vi "FPGA Main Default.vi"() -> ()   [LabVIEW 2015]
doc: "The myRIO v1.1 FPGA Shipping Personality. This personality contains support for:\n- 2 Analog Input Interrupt channel\n- 4 Digital Input Interrupt channel\n- 1 Timer\n- 1 Accelerometer\n- 1 Button\n- 4 LED\n- 10 Analog Input channels with 1 Sample\n- 6 Analog Output channels with 1 Sample\n- 40 Digital I/O channels with 1 Sample\n- 2 I2C channels\n- 4 Encoder channels\n- 6 PWM channels\n- 2 SPI channels"
uses:
  Sub VIs/Utilities/Start Boolean.ctl
  <vilib>/Platform/TimedLoop/XDataNode/timing_clust.ctl
  <vilib>/Platform/TimedLoop/XDataNode/nitl_modes.ctl
  <vilib>/Platform/TimedLoop/XDataNode/wakeup.ctl
  <vilib>/rvi/Emulation/niFpgaGetClockAttributes.vi
  <vilib>/rvi/Emulation/niFpgaSctlEmulationGetInTimedLoop.vi
  <vilib>/rvi/Emulation/niFpgaEmulationReportErrorSimple.vi
  <vilib>/rvi/eio/common/nirviEmuTemplateMethod_errors.vi
  <vilib>/rvi/Emulation/niFpgaCriticalErrorInLSC.vi
  <vilib>/rvi/Emulation/niFpgaProcessEmulError.vi
  <vilib>/rvi/Emulation/niFpgaEmulationIsFPGAContextNoSignature.vi
  <vilib>/rvi/errors/niFpgaSetErrorForExecOnDevCompSimple.vi
  <vilib>/rvi/eio/common/nirviEmuReportErrorAndStop.vi
  <vilib>/rvi/DataTransferAndStorage/Container/Common/niFpgaContainerGetUniqueNameForEmu.vi
  <vilib>/rvi/FIFO/Fifo_Resource/nirvififoEmulationSetSize.vi
  <vilib>/rvi/FIFO/Fifo_Resource/nirviFifoEmulationQueueMgr.vi
  <instcachedir>/0/nirviFifoEmulationQueueMgr_E5CAEC123FF24DC58D834DCA3CDAA9B5.lvgen/nirviFifoEmulationQueueMgr_E5CAEC123FF24DC58D834DCA3CDAA9B5_002.vi
  <vilib>/rvi/FIFO/Fifo_Resource/nirvififoEmulationDetermineInputValidOut.vi
  <vilib>/rvi/FIFO/Fifo_Resource/nirvififoEmulationCreateLock.vi
  <vilib>/rvi/FIFO/Fifo_Resource/nirvififoEmulationObtainLock.vi
  <vilib>/rvi/FIFO/Fifo_Resource/nirvififoEmulationReleaseLock.vi
  <vilib>/rvi/occurrence/nirviWaitOnOccurrenceBase.vi
  <vilib>/rvi/errors/nirviReportUnexpectedCaseInternalError.vi
  <vilib>/rvi/errors/nirviReportUnexpectedCaseInternalError (U32).vi
  <vilib>/Utility/error.llb/Clear Errors.vi
  <vilib>/rvi/DataTransferAndStorage/Container/Common/niFpgaContainerSetEmuInfo.vi
  <vilib>/eio/EIONode/EIONode.xnode
  <vilib>/rvi/DataTransferAndStorage/Container/XNode/niFpgaContainer.xnode
  <vilib>/rvi/FIFO/Fifo_Resource/nirvififoEmulationWrite.vi
  <vilib>/rvi/FIFO/Fifo_Resource/nirvififoEmulationRead.vi
  <vilib>/Platform/TimedLoop/XDataNode/XDataNode.xnode
  <vilib>/rvi/LocalResourceManager/LocalResourceManager.xnode
  <vilib>/Platform/TimedLoop/XDataNode/XDNodeRunTimeDep.lvlib
panel:
  in  "AO.A_0.VAL":u16
  in  "AO.A_1.VAL":u16
  in  "AO.B_0.VAL":u16
  in  "AO.B_1.VAL":u16
  out "AI.B_3.VAL":u16
  out "AI.B_2.VAL":u16
  out "AI.B_1.VAL":u16
  out "AI.B_0.VAL":u16
  out "AI.A_3.VAL":u16
  out "AI.A_2.VAL":u16
  out "AI.A_1.VAL":u16
  out "AI.A_0.VAL":u16
  out "DIO.B_7:0.IN":u8 format="%08b"
  in  "DIO.B_7:0.DIR":u8 format="%08b"
  in  "DIO.B_7:0.OUT":u8 format="%08b"
  in  "PWM.A_2.CS":u8=1
  in  "PWM.A_2.CNFG":u8=4
  out "PWM.A_2.CNTR":u16
  in  "PWM.A_2.MAX":u16=39999
  in  "PWM.A_2.CMP":u16=20000
  in  "PWM.A_1.CS":u8=1
  in  "PWM.A_1.CNFG":u8=4
  out "PWM.A_1.CNTR":u16
  in  "PWM.A_1.MAX":u16=39999
  in  "PWM.A_1.CMP":u16=20000
  in  "PWM.A_0.CS":u8=1
  in  "PWM.A_0.CNFG":u8=4
  out "PWM.A_0.CNTR":u16
  in  "PWM.A_0.CMP":u16=20000
  in  "PWM.A_0.MAX":u16=39999
  in  "SPI.A.DATO":u16
  out "SPI.A.DATI":u16
  in  "SPI.A.CNFG":u16=112
  in  "SPI.A.CNT":u16=19
  in  "SPI.B.CNT":u16=19
  in  "SPI.B.CNFG":u16=112 format="%0.0f"
  out "SPI.B.DATI":u16
  in  "SPI.B.DATO":u16
  in  "ENC.A.CNFG":u8 format="%08b"
  in  "ENC.B.CNFG":u8 format="%08b"
  out "ENC.A.CNTR":u32
  out "ENC.B.CNTR":u32
  out "ENC.A.STAT":u8 format="%08b"
  out "ENC.B.STAT":u8 format="%08b"
  in  "SPI.A.GO":T1
  out "SPI.A.STAT":u8 format="%08b"
  in  "SPI.B.GO":T1
  out "SPI.B.STAT":u8 format="%08b"
  out "I2C.B.STAT":u8 format="%08b"
  in  "I2C.B.CNTL":u8 format="%08b"
  out "I2C.A.STAT":u8 format="%08b"
  in  "I2C.A.CNTL":u8 format="%08b"
  in  "I2C.B.CNTR":u8=213
  in  "I2C.B.ADDR":u8 format="%08.0f"
  out "I2C.B.DATI":u8
  in  "I2C.B.DATO":u8
  in  "I2C.A.CNTR":u8=213
  in  "I2C.A.ADDR":u8 format="%08b"
  out "I2C.A.DATI":u8
  in  "I2C.A.DATO":u8
  in  "I2C.B.CNFG":u8=1 format="%08b"
  in  "I2C.A.CNFG":u8=1 format="%08b"
  in  "I2C.A.GO":T1
  in  "I2C.B.GO":T1
  out "SYS.AI.RDY":bool
  out "SYS.RDY":bool
  in  "PWM.B_2.CS":u8=1
  in  "PWM.B_2.CNFG":u8=4
  out "PWM.B_2.CNTR":u16
  in  "PWM.B_2.MAX":u16=39999
  in  "PWM.B_2.CMP":u16=20000
  in  "PWM.B_1.CS":u8=1
  in  "PWM.B_1.CNFG":u8=4
  out "PWM.B_1.CNTR":u16
  in  "PWM.B_1.MAX":u16=39999
  in  "PWM.B_1.CMP":u16=20000
  in  "PWM.B_0.CS":u8=1
  in  "PWM.B_0.CNFG":u8=4
  out "PWM.B_0.CNTR":u16
  in  "PWM.B_0.MAX":u16=39999
  in  "PWM.B_0.CMP":u16=20000
  out "DIO.A_7:0.IN":u8 format="%08b"
  in  "DIO.A_7:0.OUT":u8 format="%08b"
  in  "DIO.A_7:0.DIR":u8 format="%08b"
  in  "SYS.SELECTB":u8 format="%08b"
  in  "SYS.SELECTA":u8 format="%08b"
  out "DIO.A_15:8.IN":u8 format="%08b"
  in  "DIO.A_15:8.OUT":u8 format="%08b"
  in  "DIO.A_15:8.DIR":u8 format="%08b"
  out "DIO.B_15:8.IN":u8 format="%08b"
  in  "DIO.B_15:8.DIR":u8 format="%08b"
  in  "DIO.B_15:8.OUT":u8 format="%08b"
  in  "AO.SYS.GO":T1
  out "ACC.X.VAL":u16
  out "ACC.Y.VAL":u16
  out "SYS.ACC.RDY":bool
  out "ACC.Z.VAL":u16
  in  "DO.LED3:0":u8 format="%04b"
  out "DI.BTN":u8 format="%08b"
  out "AO.SYS.STAT":bool
  in  "IRQ.AI_A_3:0.CNFG":u8 format="%.0b"
  in  "IRQ.AI_A_0.THRESHOLD":u16
  in  "IRQ.AI_A_1.THRESHOLD":u16
  in  "IRQ.AI_A_0.NO":u8
  in  "IRQ.AI_A_1.NO":u8
  in  "IRQ.DIO_A_7:0.ENA":u8 format="%08b"
  in  "IRQ.DIO_A_7:0.RISE":u8 format="%08b"
  in  "IRQ.DIO_A_7:0.FALL":u8 format="%08b"
  in  "IRQ.DIO_A_0.NO":u8
  in  "IRQ.DIO_A_1.NO":u8
  in  "IRQ.DIO_A_2.NO":u8
  in  "IRQ.DIO_A_3.NO":u8
  in  "IRQ.DIO_A_3.CNT":u32
  in  "IRQ.DIO_A_2.CNT":u32
  in  "IRQ.DIO_A_1.CNT":u32
  in  "IRQ.DIO_A_0.CNT":u32
  in  "IRQ.AI_A_1.HYSTERESIS":u16=17
  in  "IRQ.TIMER.WRITE":u32
  in  "IRQ.TIMER.SETTIME":T1
  out "IRQ.TIMER.READ":u32
  in  "SPI.A.IRQ.NO":u8=15
  in  "SPI.B.IRQ.NO":u8=15
  in  "IRQ.AI_A_0.HYSTERESIS":u16=17
  in  "IRQ.DI_BTN.ENA":bool
  in  "IRQ.DI_BTN.RISE":bool
  in  "IRQ.DI_BTN.FALL":bool
  in  "IRQ.DI_BTN.CNT":u32
  in  "IRQ.DI_BTN.NO":u8
  # "System"
  # "Onboard Devices"
  # "Connector A"
  # "Connector B"
  # "Accelerometer"
  # "Analog Input"
  # "Analog Output"
  # "Digital I/O"
  # "PWM"
  # "SPI Master"
  # "Analog Input"
  # "Analog Output"
  # "Digital I/O"
  # "PWM"
  # "SPI Master"
  # "IO Configuration"
  # "IO Configuration"
  # "Buttons & LEDs"
  # "Analog Interrupt"
  # "Digital Interrupt"
  # "Encoders"
  # "Encoders"
  # "Button Interrupt"
  # "I2C Master"
  # "I2C Master"
  # "Timer Interrupt"
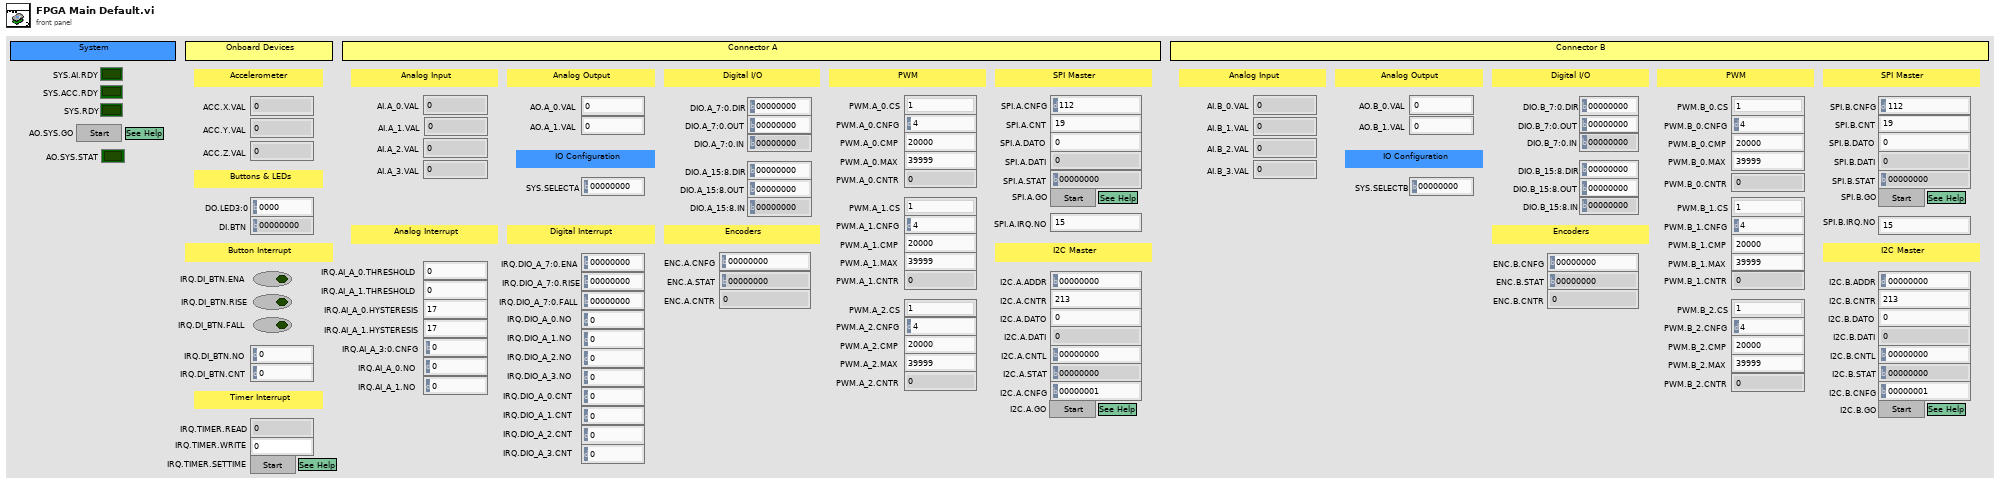
[diagram p1: front panel]
types:
  T1 = typedef "Start Boolean.ctl" = bool
  T2 = typedef "XDNodeRunTimeDep.lvlib/timing_clust.ctl" = cluster{"Expected End [f-1]":u64, "Actual End [f-1]":u64, "Finished Late? [f-1]":bool, "Expected End [i-1]":u64, "Actual End [i-1]":u64, "Finished Late? [i-1]":bool, "Expected Start [i]":u64, "Actual Start [i]":u64, "Expected Start [f]":u64, "Actual Start [f]":u64, "Source Name":string, "Structure Name":string, "Period":i64, "Deadline":i64, "Offset":i64, "Start":i64, "Priority":i32, "Timeout":i32, "Mode":T3, "Wakeup Reason":T4, "Error":errorcluster, "Source Type":string, "Secondary Source Type":string, "Global End Time":u64, "Global Start Time":u64, "Frame Duration":u64, "Iteration Duration":u64, "Assigned CPU":i32, "I/O Scan Engine Mode":u32}
  T3 = typedef "XDNodeRunTimeDep.lvlib/nitl_modes.ctl" = enum32{"No Change", "Process missed periods, maintain original phase", "Discard missed periods, maintain original phase", "Process missed periods, ignore original phase", "Discard missed periods, ignore original phase"}
  T4 = typedef "XDNodeRunTimeDep.lvlib/wakeup.ctl" = enum32{"Normal", "Aborted", "Asynchronous wakeup", "Timing source error", "Timed loop error", "Timeout"}
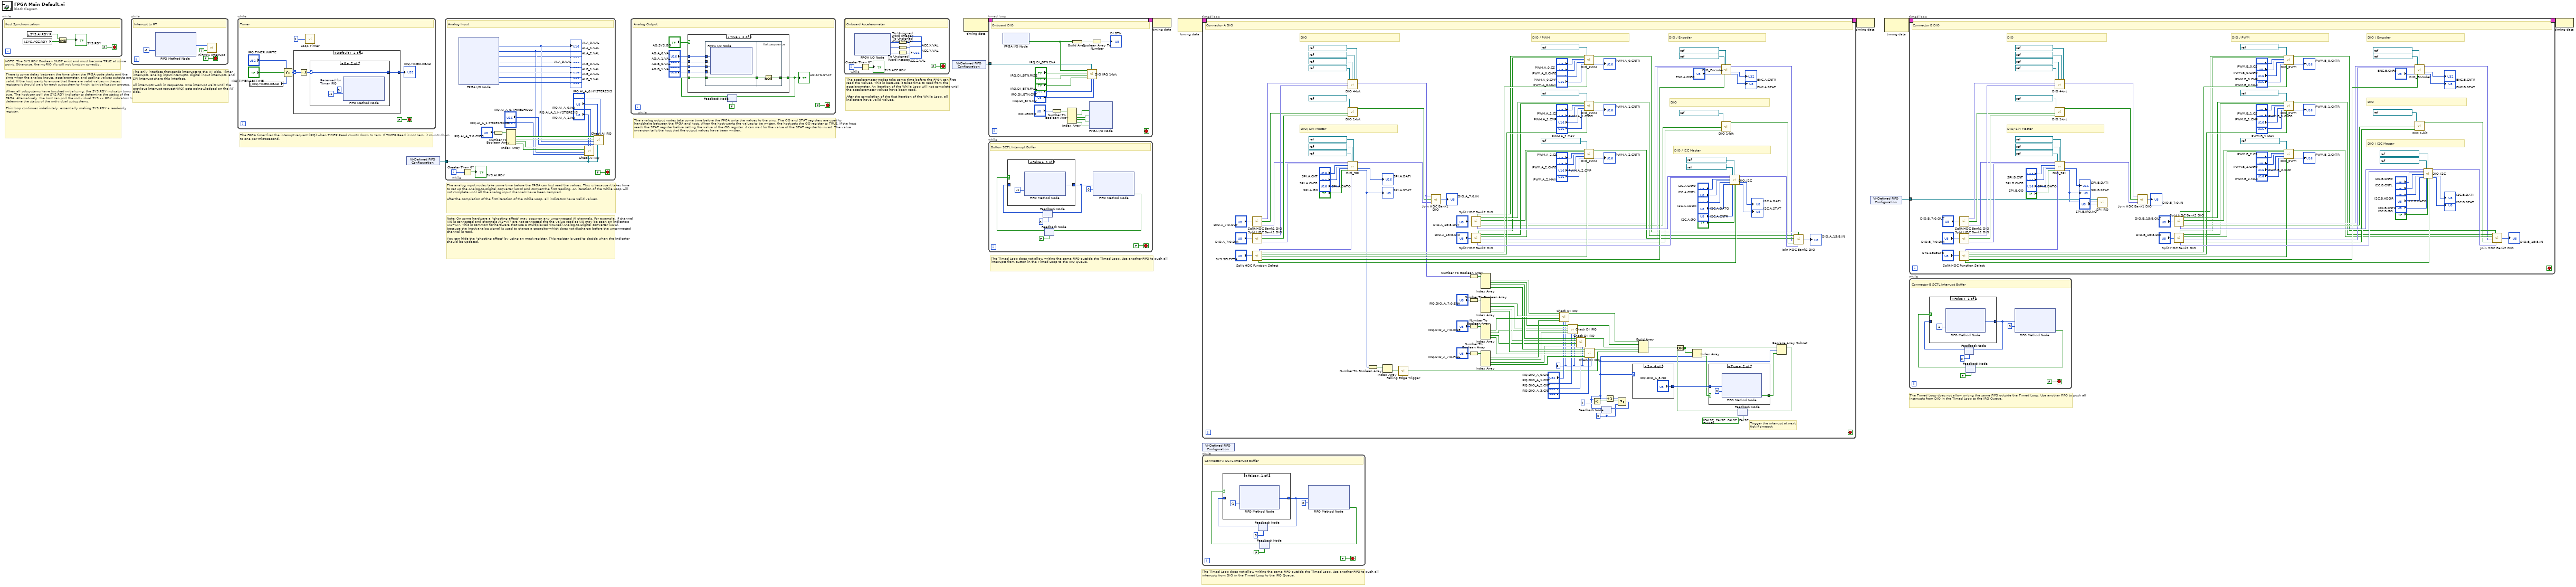
[diagram p0: block diagram]
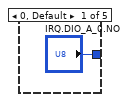
[diagram p9: hidden frame]
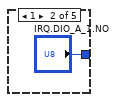
[diagram p10: hidden frame]
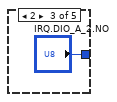
[diagram p11: hidden frame]
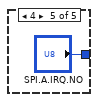
[diagram p12: hidden frame]
diagram:
  # "The Timed Loop does not allow writing the same FIFO outside the Timed Loop. Use another FIFO to push all interrupts from DIO in the Timed Loop to the IRQ Queue."
  # "The Timed Loop does not allow writing the same FIFO outside the Timed Loop. Use another FIFO to push all interrupts from DIO in the Timed Loop to the IRQ Queue."
  # "The Timed Loop does not allow writing the same FIFO outside the Timed Loop. Use another FIFO to push all interrupts from Button in the Timed Loop to the IRQ Queue."
  # "The accelerometer nodes take some time before the FPGA can first read the values. This is because it takes time to read from the accelerometer. An iteration of the While Loop will not complete until the accelerometer values have been read.\n\nAfter the completion of the first iteration of the While Loop, all indicators have valid values."
  # "The analog output nodes take some time before the FPGA write the values to the pins. The GO and STAT registers are used to handshake between the FPGA and host. When the host wants the values to be written, the host sets the GO register to TRUE. If the host reads the STAT register before setting the value of the GO register, it can wait for the value of the STAT register to invert. The value inversion tells the host that the output values have been written."
  # "The analog input nodes take some time before the FPGA can first read the values. This is because it takes time to set up the Analog-to-Digital converter (ADC) and convert the first reading. An iteration of the While Loop will not complete until all the analog input channels have been sampled.\n\nAfter the completion of the first iteration of the While Loop, all indicators have valid values."
  # "Note: On some hardware a \"ghosting effect\" may occur on any unconnected AI channels. For example, if channel AI0 is connected and channels AI1~AI7 are not connected the the value read at AI0 may be seen on indicators AI1~AI7. This is common for hardware that use a multiplexed (MUXed) Analog-to-Digital converter (ADC), because the input analog signal is used to charge a capacitor which does not discharge before the unconnected channel is read.\n\nYou can hide the \"ghosting effect\" by using an mask register. This register is used to decide when the indicator should be updated."
  # "The FPGA timer fires the interrupt request (IRQ) when TIMER.Read counts down to zero. If TIMER.Read is not zero, it counts down to one per microsecond."
  # "The only interface that sends interrupts to the RT side. Timer interrupts, analog input interrupts, digital input interrupts, and SPI interrupt share this interface.\n\nAll interrupts work in sequence. One interrupt waits until the previous interrupt request (IRQ) gets acknowledged on the RT side."
  # "NOTE: The SYS.RDY Boolean MUST exist and must become TRUE at some point. Otherwise, the myRIO VIs will not function correctly."
  # "There is some delay between the time when the FPGA code starts and the time when the analog inputs, accelerometer, and scaling values outputs are valid. If the host wants to ensure that there are valid values in theses registers it should wait for each subsystem to finish its initialization process. \n\nWhen all subsystems have finished initializinig, the SYS.RDY indicator turns true. The host can poll the SYS.RDY indicator to determine the status of the FPGA. Alternatively, the host can poll the individual SYS.xx.RDY indicators to determine the status of the individual subsystems.\n\nThis loop continues indefinitely, essentially making SYS.RDY a read-only register."
  n1 = while {
    stop <- FALSE stop-if-true
    # "Host Synchronization"
    n2 = local read "SYS.ACC.RDY"() -> (w11:bool)
    n3 = local read "SYS.AI.RDY"() -> (w13:bool)
    n4 = Compound Arithmetic op=AND(w13, w11) -> (→"SYS.RDY":bool)
  }
  n5 = while {
    stop <- FALSE stop-if-true
    # "Interrupt to RT"
    n6 = xnode ("FIFO Method Node")("Timeout"=-1) -> ("Element"=w16:u8)  [unwired: 1 in, 2 out]
    n7 = call <vilib>:"niFPGA Interrupt.vi"("Wait Until Cleared (F)"=TRUE, "IRQ Number (0)"=w16) -> ()  [unwired: 1 in]
  }
  n8 = while {
    stop <- FALSE stop-if-true
    # "Timer"
    n9 = local read "IRQ.TIMER.READ"() -> (w21:u32)
    n10 = Select(t="IRQ.TIMER.WRITE", s="IRQ.TIMER.SETTIME", f=w21) -> (s? t:f=w19:u32)
    n11 = case shown="Default" w19 {
      selector: w19 -> [w25 w28]
      tunnel: [w25 w26] -> w18
      frame 0 {
      }
      frame Default {
        n12 = Decrement(x=w28) -> (x-1=w27:u32)
        n13 = case shown="0" w27 {
          selector: w27 -> [w29 w32]
          tunnel: [w29 w32] -> w26
          frame Default {
          }
          frame 0 {
            w31 = u8 0  # Reserved for Timer IRQ
            n14 = xnode ("FIFO Method Node")("Element"=w31, "Timeout"=-1) -> ()  [unwired: 1 in, 2 out]
          }
        }
      }
    }
    "IRQ.TIMER.READ" <- w18
    n15 = call "Loop Timer"("Count(uSec)"=u8 1 ("Count(mSec)")) -> ()  [unwired: 1 out]
  }
  n16 = xnode "VI-Defined FIFO Configuration"() -> ("FIFO Out"=w3:refnum<k21>)
  n17 = while {
    tunnel: w3 -> [w34]
    i -> [w53]
    stop <- FALSE stop-if-true
    # "Analog Input"
    n18 = xnode "FPGA I/O Node"() -> ("ConnectorA/AI0"=w39:u16, "ConnectorA/AI1"=w38:u16, "ConnectorA/AI2"=→"AI.A_2.VAL":u16, "ConnectorA/AI3"=→"AI.A_3.VAL":u16, "ConnectorB/AI0"=→"AI.B_0.VAL":u16, "ConnectorB/AI1"=→"AI.B_1.VAL":u16, "ConnectorB/AI2"=→"AI.B_2.VAL":u16, "ConnectorB/AI3"=→"AI.B_3.VAL":u16)  [unwired: 8 in, 8 out]
    "AI.A_0.VAL" <- w39
    "AI.A_1.VAL" <- w38
    n19 = Greater Than 0?(x=w53) -> (x > 0?=→"SYS.AI.RDY":bool)
    n20 = Number To Boolean Array(number="IRQ.AI_A_3:0.CNFG") -> (Boolean array=w49:bool[])
    n21 = Index Array(array=w49) -> (element #1=w47:bool, element #2=w46:bool, element #3=w44:bool, element #4=w43:bool)  [unwired: 4 in]
    n22 = call "Check AI IRQ.vi"("Hysteresis"="IRQ.AI_A_1.HYSTERESIS", "FIFO In"=w34, "IRQ Number"="IRQ.AI_A_1.NO", "Threshold"="IRQ.AI_A_1.THRESHOLD", "Analog Value"=w38, "Rising Edge?"=w43, "Enable Interrupt?"=w44) -> ()  [unwired: 5 in]
    n23 = call "Check AI IRQ.vi"("Hysteresis"="IRQ.AI_A_0.HYSTERESIS", "FIFO In"=w34, "IRQ Number"="IRQ.AI_A_0.NO", "Threshold"="IRQ.AI_A_0.THRESHOLD", "Analog Value"=w39, "Rising Edge?"=w46, "Enable Interrupt?"=w47) -> ()  [unwired: 5 in]
  }
  n24 = while {
    stop <- FALSE stop-if-true
    # "Analog Output"
    n25 = feedback #1(FALSE) -> (w59:bool)
    n26 = case shown="True" "AO.SYS.GO" {
      tunnel: "AO.A_0.VAL" -> [_ w73]
      tunnel: "AO.A_1.VAL" -> [_ w72]
      tunnel: "AO.B_0.VAL" -> [_ w71]
      tunnel: "AO.B_1.VAL" -> [_ w70]
      tunnel: w59 -> [w66 w69]
      tunnel: [w66 w67] -> w57
      frame False {
      }
      frame True {
        n27 = flat-sequence {
          tunnel: w73 -> [w78]
          tunnel: w72 -> [w77]
          tunnel: w71 -> [w76]
          tunnel: w70 -> [w75]
          tunnel: w69 -> [w74]
          tunnel: [w74] -> w68
          tunnel: w68 -> [w80]
          tunnel: [w79] -> w67
          frame #0 {
            n28 = xnode "FPGA I/O Node"("ConnectorA/AO0"=w78, "ConnectorA/AO1"=w77, "ConnectorB/AO0"=w76, "ConnectorB/AO1"=w75) -> ()  [unwired: 4 in, 4 out]
          }
          frame #1 {
            n29 = Not(x=w80) -> (.not. x?=w79:bool)
          }
        }
      }
    }
    "AO.SYS.STAT" <- w57
    n30 = feedback-in #1(w57) -> ()
  }
  n31 = while {
    i -> [w85]
    stop <- FALSE stop-if-true
    # "Onboard Accelerometer"
    n32 = xnode "FPGA I/O Node"() -> ("AccelerationX"=w88:i16, "AccelerationY"=w87:i16, "AccelerationZ"=w86:i16)  [unwired: 3 in, 3 out]
    n33 = Greater Than 0?(x=w85) -> (x > 0?=→"SYS.ACC.RDY":bool)
    n34 = To Unsigned Word Integer(number=w88) -> (unsigned 16bit integer=→"ACC.X.VAL":u16)
    n35 = To Unsigned Word Integer(number=w87) -> (unsigned 16bit integer=→"ACC.Y.VAL":u16)
    n36 = To Unsigned Word Integer(number=w86) -> (unsigned 16bit integer=→"ACC.Z.VAL":u16)
  }
  n37 = xnode "VI-Defined FIFO Configuration"() -> ("FIFO Out"=w2:refnum<k21>)
  n38 = node-c288() -> (w5:T2)  [unwired: 1 in]
  n39 = timed-loop {
    timing: w5 -> [_]
    timing-out: [_] -> w4
    tunnel: w2 -> [w90]
    stop <- _ stop-if-true
    # "Onboard DIO"
    n40 = xnode "FPGA I/O Node"() -> ("Button0"=w96:bool)  [unwired: 1 in, 1 out]
    n41 = Number To Boolean Array(number="DO.LED3:0") -> (Boolean array=w101:bool[])
    n42 = Index Array(array=w101) -> (element #1=w100:bool, element #2=w99:bool, element #3=w98:bool, element #4=w97:bool)  [unwired: 4 in]
    n43 = Build Array(w96) -> (w104:bool[])
    n44 = call "DIO IRQ 1-bit.vi"("IRQ.NO"="IRQ.DI_BTN.NO", "IRQ.CNT"="IRQ.DI_BTN.CNT", "FIFO in"=w90, "IRQ.FALL"="IRQ.DI_BTN.FALL", "IRQ.RISE"="IRQ.DI_BTN.RISE", "IRQ.ENA"="IRQ.DI_BTN.ENA", "DIO"=w96) -> ()  [unwired: 5 in]
    n45 = xnode "FPGA I/O Node"("LED0"=w100, "LED1"=w99, "LED2"=w98, "LED3"=w97) -> ()  [unwired: 4 in, 4 out]
    n46 = Boolean Array To Number(Boolean array=w104) -> (number=→"DI.BTN":u8)
  }
  n47 = while {
    stop <- FALSE stop-if-true
    # "Button SCTL Interrupt Buffer"
    n48 = feedback #2(u8 0 ("Element")) -> (w109:u8)
    n49 = feedback #3(FALSE ("Timed Out?")) -> (w113:bool)
    n50 = case shown="False" w113 {
      tunnel: [w115 w117] -> w110
      tunnel: w109 -> [_ w117]
      frame False {
        n51 = xnode ("FIFO Method Node")("Timeout"=-1) -> ("Element"=w115:u8)  [unwired: 1 in, 2 out]
      }
      frame True {
      }
    }
    n52 = feedback-in #2(w110) -> ()
    n53 = xnode ("FIFO Method Node")("Element"=w110, "Timeout"=0) -> ("Timed Out?"=w111:bool)  [unwired: 1 in, 1 out]
    n54 = feedback-in #3(w111) -> ()
  }
  n55 = node-c288(w4) -> ()
  n56 = node-c288() -> (w9:T2)  [unwired: 1 in]
  n57 = xnode "VI-Defined FIFO Configuration"() -> ()  [unwired: 1 out]
  n58 = while {
    stop <- FALSE stop-if-true
    # "Connector A SCTL Interrupt Buffer"
    n59 = feedback #4(u8 0 ("Element")) -> (w120:u8)
    n60 = feedback #5(FALSE ("Timed Out?")) -> (w124:bool)
    n61 = case shown="False" w124 {
      tunnel: [w126 w128] -> w121
      tunnel: w120 -> [_ w128]
      frame False {
        n62 = xnode ("FIFO Method Node")("Timeout"=-1) -> ("Element"=w126:u8)  [unwired: 1 in, 2 out]
      }
      frame True {
      }
    }
    n63 = feedback-in #4(w121) -> ()
    n64 = xnode ("FIFO Method Node")("Element"=w121, "Timeout"=0) -> ("Timed Out?"=w122:bool)  [unwired: 1 in, 1 out]
    n65 = feedback-in #5(w122) -> ()
  }
  n66 = timed-loop {
    timing: w9 -> [_]
    timing-out: [_] -> w8
    stop <- _ stop-if-true
    w129 = u16 5 ("Debounce Ticks")
    w130 = u8 0
    # "Trigger the interrupt at next \ntick if timeout"
    # "DIO / Encoder"
    # "DIO / I2C Master"
    # "DIO / PWM"
    # "DIO"
    # "DIO"
    # "DIO/ SPI Master"
    # "Connector A DIO"
    n67 = call "Split HDC Bank1 DIO.vi"("IN 7:0"="DIO.A_7:0.OUT") -> ("OUT 3:0"=w265:fxp<+,4,4>, "OUT 4"=w184:bool, "OUT 7:5"=w262:fxp<+,3,3>)
    n68 = call "Split HDC Bank1 DIO.vi"("IN 7:0"="DIO.A_7:0.DIR") -> ("OUT 3:0"=w264:fxp<+,4,4>, "OUT 4"=w263:bool, "OUT 7:5"=w261:fxp<+,3,3>)
    n69 = call "Split HDC Function Select.vi"("IN 7:0"="SYS.SELECTA") -> ("OUT 1:0"=w204:fxp<+,2,2>, "OUT 7"=w199:bool, "OUT 2"=w203:bool, "OUT 3"=w202:bool, "OUT 4"=w201:bool, "OUT 5"=w200:bool)
    n70 = call "DIO 4-bit.vi"("DIO0 Refnum"=refnum<k21> "ConnectorA/DIO0", "DIO1 Refnum"=refnum<k21> "ConnectorA/DIO1", "DIO2 Refnum"=refnum<k21> "ConnectorA/DIO2", "DIR 3:0"=w264, "OUT 3:0"=w265, "DIO3 Refnum"=refnum<k21> "ConnectorA/DIO3") -> ("IN 3:0"=w152:fxp<+,4,4>)  [unwired: 5 in]
    n71 = call "DIO 1-bit.vi"("DIR"=w263, "OUT"=w184, "DIO Refnum"=refnum<k21> "ConnectorA/DIO4") -> ("IN"=w151:bool)  [unwired: 8 in]
    n72 = call "DIO_SPI.vi"("DIO.2:0.OUT"=w262, "DIO.2:0.DIR"=w261, "SPI.CNT"="SPI.A.CNT", "SPI.CNFG"="SPI.A.CNFG", "SPI.DATO"="SPI.A.DATO", "SPI.GO"="SPI.A.GO", "DIO.2/SPI.MOSI Refnum"=refnum<k21> "ConnectorA/DIO7" ("DIO.2/SPI.SCLK"), "SELECT.1:0"=w204, "DIO.1/SPI.MISO Refnum"=refnum<k21> "ConnectorA/DIO6" ("DIO.1/SPI.MOSI"), "DIO.0/SPI.SCLK Refnum"=refnum<k21> "ConnectorA/DIO5" ("DIO.0/SPI.MISO")) -> ("DIO.2:0.IN"=w237:fxp<+,3,3>, "SPI.DATI"=→"SPI.A.DATI":u16, "SPI.STAT"=w137:u8)  [unwired: 7 in]
    "SPI.A.STAT" <- w137
    n73 = Number To Boolean Array(number=w137) -> (Boolean array=w139:bool[])
    n74 = Index Array(array=w139) -> (element=w138:bool)  [unwired: 1 in]
    n75 = call "Falling Edge Trigger.vi"("Signal"=w138) -> ("Trigger?"=w136:bool)
    n76 = call "Join HDC Bank1 DIO.vi"("IN 7:5"=w237, "IN 4"=w151, "IN 3:0"=w152) -> ("OUT 7:0"=→"DIO.A_7:0.IN":u8)
    n77 = Number To Boolean Array(number=w152) -> (Boolean array=w177:bool[])
    n78 = Number To Boolean Array(number="IRQ.DIO_A_7:0.ENA") -> (Boolean array=w183:bool[])
    n79 = Number To Boolean Array(number="IRQ.DIO_A_7:0.RISE") -> (Boolean array=w182:bool[])
    n80 = Number To Boolean Array(number="IRQ.DIO_A_7:0.FALL") -> (Boolean array=w181:bool[])
    n81 = call "Split HDC Bank2 DIO.vi"("IN 7:0"="DIO.A_15:8.OUT") -> ("OUT 5"=w186:bool, "OUT 7:6"=w208:fxp<+,2,2>, "OUT 4:3"=w188:fxp<+,2,2>, "OUT 2"=w190:bool, "OUT 0"=w194:bool, "OUT 1"=w193:bool)  [unwired: 2 in]
    n82 = call "Split HDC Bank2 DIO.vi"("IN 7:0"="DIO.A_15:8.DIR") -> ("OUT 5"=w185:bool, "OUT 7:6"=w207:fxp<+,2,2>, "OUT 4:3"=w187:fxp<+,2,2>, "OUT 2"=w189:bool, "OUT 0"=w192:bool, "OUT 1"=w191:bool)  [unwired: 2 in]
    n83 = Index Array(array=w177) -> (element #1=w158:bool, element #2=w173:bool, element #3=w172:bool, element #4=w171:bool)  [unwired: 4 in]
    n84 = Index Array(array=w183) -> (element #1=w176:bool, element #2=w170:bool, element #3=w169:bool, element #4=w168:bool)  [unwired: 4 in]
    n85 = Index Array(array=w182) -> (element #1=w175:bool, element #2=w167:bool, element #3=w166:bool, element #4=w165:bool)  [unwired: 4 in]
    n86 = Index Array(array=w181) -> (element #1=w174:bool, element #2=w164:bool, element #3=w163:bool, element #4=w162:bool)  [unwired: 4 in]
    n87 = call "Check DI IRQ.vi"("Debounce Ticks"=w129, "Count"="IRQ.DIO_A_0.CNT", "On Falling Edge?"=w174, "On Rising Edge?"=w175, "Enable Interrupt?"=w176, "Digital In"=w158) -> ("Trigger?"=w149:bool)  [unwired: 5 in]
    n88 = call "Check DI IRQ.vi"("Debounce Ticks"=w129, "Count"="IRQ.DIO_A_1.CNT", "On Falling Edge?"=w164, "On Rising Edge?"=w167, "Enable Interrupt?"=w170, "Digital In"=w173) -> ("Trigger?"=w148:bool)  [unwired: 5 in]
    n89 = call "Check DI IRQ.vi"("Debounce Ticks"=w129, "Count"="IRQ.DIO_A_2.CNT", "On Falling Edge?"=w163, "On Rising Edge?"=w166, "Enable Interrupt?"=w169, "Digital In"=w172) -> ("Trigger?"=w147:bool)  [unwired: 5 in]
    n90 = call "DIO_PWM.vi"("DIO.OUT"=w194, "DIO.DIR"=w192, "PWM.CS"="PWM.A_0.CS", "PWM.CNFG"="PWM.A_0.CNFG", "PWM.CMP"="PWM.A_0.CMP", "PWM.MAX"="PWM.A_0.MAX", "DIO/PWM"=refnum<k21> "ConnectorA/DIO8", "SELECT"=w203) -> ("DIO.IN"=w198:bool, "PWM.CNTR"=→"PWM.A_0.CNTR":u16)  [unwired: 10 in]
    n91 = call "DIO_PWM.vi"("DIO.OUT"=w193, "DIO.DIR"=w191, "PWM.CS"="PWM.A_1.CS", "PWM.CNFG"="PWM.A_1.CNFG", "PWM.CMP"="PWM.A_1.CMP", "PWM.MAX"="PWM.A_1.MAX", "DIO/PWM"=refnum<k21> "ConnectorA/DIO9", "SELECT"=w202) -> ("DIO.IN"=w197:bool, "PWM.CNTR"=→"PWM.A_1.CNTR":u16)  [unwired: 10 in]
    n92 = call "DIO_PWM.vi"("DIO.OUT"=w190, "DIO.DIR"=w189, "PWM.CS"="PWM.A_2.CS", "PWM.CNFG"="PWM.A_2.CNFG", "PWM.CMP"="PWM.A_2.CMP", "PWM.MAX"="PWM.A_2.MAX", "DIO/PWM"=refnum<k21> "ConnectorA/DIO10", "SELECT"=w201) -> ("DIO.IN"=w196:bool, "PWM.CNTR"=→"PWM.A_2.CNTR":u16)  [unwired: 10 in]
    n93 = call "Check DI IRQ.vi"("Debounce Ticks"=w129, "Count"="IRQ.DIO_A_3.CNT", "On Falling Edge?"=w162, "On Rising Edge?"=w165, "Enable Interrupt?"=w168, "Digital In"=w171) -> ("Trigger?"=w146:bool)  [unwired: 5 in]
    n94 = feedback #6(w130) -> (w132:u8)
    n95 = Less?(x=w132, y=4 ("x")) -> (x < y?=w134:bool)
    n96 = Increment(x=w132) -> (x+1=w133:u8)
    n97 = Select(t=w133, s=w134, f=w130) -> (s? t:f=w131:u8)
    n98 = feedback-in #6(w131) -> ()
    n99 = case shown="3" w132 {
      tunnel: ["IRQ.DIO_A_0.NO" "IRQ.DIO_A_1.NO" "IRQ.DIO_A_2.NO" "IRQ.DIO_A_3.NO" "SPI.A.IRQ.NO"] -> w161
      frame 0, Default {
      }
      frame 1 {
      }
      frame 2 {
      }
      frame 3 {
      }
      frame 4 {
      }
    }
    n100 = Build Array(w149, w148, w147, w146, w136) -> (w144:bool[])
    n101 = call "DIO_Encoder.vi"("DIO.1:0.OUT"=w188, "DIO.1:0.DIR"=w187, "QE.CNFG"="ENC.A.CNFG", "DIO.1/QE.B"=refnum<k21> "ConnectorA/DIO12", "SELECT"=w200, "DIO.0/QE.A"=refnum<k21> "ConnectorA/DIO11") -> ("DIO.1:0.IN"=w195:fxp<+,2,2>, "QE.CNTR"=→"ENC.A.CNTR":u32, "QE.STAT"=→"ENC.A.STAT":u8)  [unwired: 11 in]
    n102 = call "DIO 1-bit.vi"("DIR"=w185, "OUT"=w186, "DIO Refnum"=refnum<k21> "ConnectorA/DIO13") -> ("IN"=w150:bool)  [unwired: 8 in]
    n103 = call "DIO_I2C.vi"("DIO.1:0.OUT"=w208, "DIO.1:0.DIR"=w207, "I2C.CNFG"="I2C.A.CNFG", "I2C.CNTL"="I2C.A.CNTL", "I2C.ADDR"="I2C.A.ADDR", "I2C.DATO"="I2C.A.DATO", "DIO.1/I2C.SDA"=refnum<k21> "ConnectorA/DIO15" ("DIO.1/I2C.SCL"), "I2C.CNTR"="I2C.A.CNTR", "DIO.0/I2C.SCL"=refnum<k21> "ConnectorA/DIO14" ("DIO.0/I2C.SDA"), "Execute?"="I2C.A.GO", "SELECT"=w199) -> ("DIO.1:0.IN"=w206:fxp<+,2,2>, "I2C.DATI"=→"I2C.A.DATI":u8, "I2C.STAT"=→"I2C.A.STAT":u8)  [unwired: 6 in]
    n104 = feedback #7(bool[] [FALSE, FALSE, FALSE, FALSE, FALSE] ("initialized array")) -> (w140:bool[])
    n105 = Or(x=w144, y=w140) -> (x .or. y?=w145:bool[])
    n106 = Index Array(array=w145, index=w132) -> (element=w143:bool)
    n107 = case shown="True" w143 {
      selector: w143 -> [w266 _]
      tunnel: [w266 w267] -> w142
      tunnel: w161 -> [_ w268]
      frame False {
      }
      frame True {
        n108 = xnode ("FIFO Method Node")("Element"=w268, "Timeout"=0) -> ("Timed Out?"=w267:bool)  [unwired: 1 in, 1 out]
      }
    }
    n109 = Replace Array Subset(array=w145, new element=w142, index=w132) -> (w141:bool[])
    n110 = feedback-in #7(w141) -> ()
    n111 = call "Join HDC Bank2 DIO.vi"("IN 7:6"=w206, "IN 5"=w150, "IN 4:3"=w195, "IN 0"=w198, "IN 2"=w196, "IN 1"=w197) -> ("OUT 7:0"=→"DIO.A_15:8.IN":u8)  [unwired: 4 in]
  }
  n112 = node-c288(w8) -> ()
  n113 = xnode "VI-Defined FIFO Configuration"() -> ("FIFO Out"=w1:refnum<k21>)
  n114 = node-c288() -> (w7:T2)  [unwired: 1 in]
  n115 = timed-loop {
    timing: w7 -> [_]
    timing-out: [_] -> w6
    tunnel: w1 -> [w278]
    stop <- _ stop-if-true
    # "DIO / Encoder"
    # "DIO / I2C Master"
    # "DIO / PWM"
    # "DIO"
    # "DIO"
    # "DIO/ SPI Master"
    # "Connector B DIO"
    n116 = call "Split HDC Bank1 DIO.vi"("IN 7:0"="DIO.B_7:0.OUT") -> ("OUT 3:0"=w366:fxp<+,4,4>, "OUT 4"=w364:bool, "OUT 7:5"=w362:fxp<+,3,3>)
    n117 = call "Split HDC Bank1 DIO.vi"("IN 7:0"="DIO.B_7:0.DIR") -> ("OUT 3:0"=w365:fxp<+,4,4>, "OUT 4"=w363:bool, "OUT 7:5"=w361:fxp<+,3,3>)
    n118 = call "Split HDC Function Select.vi"("IN 7:0"="SYS.SELECTB") -> ("OUT 1:0"=w338:fxp<+,2,2>, "OUT 7"=w333:bool, "OUT 2"=w337:bool, "OUT 3"=w336:bool, "OUT 4"=w335:bool, "OUT 5"=w334:bool)
    n119 = call "DIO 4-bit.vi"("DIO0 Refnum"=refnum<k21> "ConnectorB/DIO0", "DIO1 Refnum"=refnum<k21> "ConnectorB/DIO1", "DIO2 Refnum"=refnum<k21> "ConnectorB/DIO2", "DIR 3:0"=w365, "OUT 3:0"=w366, "DIO3 Refnum"=refnum<k21> "ConnectorB/DIO3") -> ("IN 3:0"=w344:fxp<+,4,4>)  [unwired: 5 in]
    n120 = call "DIO 1-bit.vi"("DIR"=w363, "OUT"=w364, "DIO Refnum"=refnum<k21> "ConnectorB/DIO4") -> ("IN"=w343:bool)  [unwired: 8 in]
    n121 = call "DIO_SPI.vi"("DIO.2:0.OUT"=w362, "DIO.2:0.DIR"=w361, "SPI.CNT"="SPI.B.CNT", "SPI.CNFG"="SPI.B.CNFG", "SPI.DATO"="SPI.B.DATO", "SPI.GO"="SPI.B.GO", "DIO.2/SPI.MOSI Refnum"=refnum<k21> "ConnectorB/DIO7" ("DIO.2/SPI.SCLK"), "SELECT.1:0"=w338, "DIO.1/SPI.MISO Refnum"=refnum<k21> "ConnectorB/DIO6" ("DIO.1/SPI.MOSI"), "DIO.0/SPI.SCLK Refnum"=refnum<k21> "ConnectorB/DIO5" ("DIO.0/SPI.MISO")) -> ("DIO.2:0.IN"=w342:fxp<+,3,3>, "SPI.DATI"=→"SPI.B.DATI":u16, "SPI.STAT"=w277:u8)  [unwired: 7 in]
    "SPI.B.STAT" <- w277
    n122 = call "SPI IRQ.vi"("SPI.A.IRQ.NO"="SPI.B.IRQ.NO", "SPI.STAT"=w277, "FIFO In"=w278) -> ()  [unwired: 9 in]
    n123 = call "Join HDC Bank1 DIO.vi"("IN 7:5"=w342, "IN 4"=w343, "IN 3:0"=w344) -> ("OUT 7:0"=→"DIO.B_7:0.IN":u8)
    n124 = call "Split HDC Bank2 DIO.vi"("IN 7:0"="DIO.B_15:8.OUT") -> ("OUT 5"=w290:bool, "OUT 7:6"=w341:fxp<+,2,2>, "OUT 4:3"=w291:fxp<+,2,2>, "OUT 2"=w292:bool, "OUT 0"=w294:bool, "OUT 1"=w293:bool)  [unwired: 2 in]
    n125 = call "Split HDC Bank2 DIO.vi"("IN 7:0"="DIO.B_15:8.DIR") -> ("OUT 5"=w285:bool, "OUT 7:6"=w340:fxp<+,2,2>, "OUT 4:3"=w286:fxp<+,2,2>, "OUT 2"=w287:bool, "OUT 0"=w289:bool, "OUT 1"=w288:bool)  [unwired: 2 in]
    n126 = call "DIO_PWM.vi"("DIO.OUT"=w294, "DIO.DIR"=w289, "PWM.CS"="PWM.B_0.CS", "PWM.CNFG"="PWM.B_0.CNFG", "PWM.CMP"="PWM.B_0.CMP", "PWM.MAX"="PWM.B_0.MAX", "DIO/PWM"=refnum<k21> "ConnectorB/DIO8", "SELECT"=w337) -> ("DIO.IN"=w284:bool, "PWM.CNTR"=→"PWM.B_0.CNTR":u16)  [unwired: 10 in]
    n127 = call "DIO_PWM.vi"("DIO.OUT"=w293, "DIO.DIR"=w288, "PWM.CS"="PWM.B_1.CS", "PWM.CNFG"="PWM.B_1.CNFG", "PWM.CMP"="PWM.B_1.CMP", "PWM.MAX"="PWM.B_1.MAX", "DIO/PWM"=refnum<k21> "ConnectorB/DIO9", "SELECT"=w336) -> ("DIO.IN"=w283:bool, "PWM.CNTR"=→"PWM.B_1.CNTR":u16)  [unwired: 10 in]
    n128 = call "DIO_PWM.vi"("DIO.OUT"=w292, "DIO.DIR"=w287, "PWM.CS"="PWM.B_2.CS", "PWM.CNFG"="PWM.B_2.CNFG", "PWM.CMP"="PWM.B_2.CMP", "PWM.MAX"="PWM.B_2.MAX", "DIO/PWM"=refnum<k21> "ConnectorB/DIO10", "SELECT"=w335) -> ("DIO.IN"=w282:bool, "PWM.CNTR"=→"PWM.B_2.CNTR":u16)  [unwired: 10 in]
    n129 = call "DIO_Encoder.vi"("DIO.1:0.OUT"=w291, "DIO.1:0.DIR"=w286, "QE.CNFG"="ENC.B.CNFG", "DIO.1/QE.B"=refnum<k21> "ConnectorB/DIO12", "SELECT"=w334, "DIO.0/QE.A"=refnum<k21> "ConnectorB/DIO11") -> ("DIO.1:0.IN"=w281:fxp<+,2,2>, "QE.CNTR"=→"ENC.B.CNTR":u32, "QE.STAT"=→"ENC.B.STAT":u8)  [unwired: 11 in]
    n130 = call "DIO 1-bit.vi"("DIR"=w285, "OUT"=w290, "DIO Refnum"=refnum<k21> "ConnectorB/DIO13") -> ("IN"=w280:bool)  [unwired: 8 in]
    n131 = call "DIO_I2C.vi"("DIO.1:0.OUT"=w341, "DIO.1:0.DIR"=w340, "I2C.CNFG"="I2C.B.CNFG", "I2C.CNTL"="I2C.B.CNTL", "I2C.ADDR"="I2C.B.ADDR", "I2C.DATO"="I2C.B.DATO", "DIO.1/I2C.SDA"=refnum<k21> "ConnectorB/DIO15" ("DIO.1/I2C.SCL"), "I2C.CNTR"="I2C.B.CNTR", "DIO.0/I2C.SCL"=refnum<k21> "ConnectorB/DIO14" ("DIO.0/I2C.SDA"), "Execute?"="I2C.B.GO", "SELECT"=w333) -> ("DIO.1:0.IN"=w339:fxp<+,2,2>, "I2C.DATI"=→"I2C.B.DATI":u8, "I2C.STAT"=→"I2C.B.STAT":u8)  [unwired: 6 in]
    n132 = call "Join HDC Bank2 DIO.vi"("IN 7:6"=w339, "IN 5"=w280, "IN 4:3"=w281, "IN 0"=w284, "IN 2"=w282, "IN 1"=w283) -> ("OUT 7:0"=→"DIO.B_15:8.IN":u8)  [unwired: 4 in]
  }
  n133 = while {
    stop <- FALSE stop-if-true
    # "Connector B SCTL Interrupt Buffer"
    n134 = feedback #8(u8 0 ("Element")) -> (w371:u8)
    n135 = feedback #9(FALSE ("Timed Out?")) -> (w375:bool)
    n136 = case shown="False" w375 {
      tunnel: [w377 w379] -> w372
      tunnel: w371 -> [_ w379]
      frame False {
        n137 = xnode ("FIFO Method Node")("Timeout"=-1) -> ("Element"=w377:u8)  [unwired: 1 in, 2 out]
      }
      frame True {
      }
    }
    n138 = feedback-in #8(w372) -> ()
    n139 = xnode ("FIFO Method Node")("Element"=w372, "Timeout"=0) -> ("Timed Out?"=w373:bool)  [unwired: 1 in, 1 out]
    n140 = feedback-in #9(w373) -> ()
  }
  n141 = node-c288(w6) -> ()
